vi "Format Header.vi"(5 "Name":string[](array[string]), 7 "Value":string[](array[string]), 11 "IPersist in":refnum<class "IPersist.lvclass">) -> (3 "IPersist out":refnum<class "IPersist.lvclass">, 4 "Header":string)   [LabVIEW 2019, in "IPersist.lvlib" / "IPersist.lvclass"]
uses:
  <vilib>/gpm_packages/@cs/persistence/source/IPersist/IPersist.lvclass
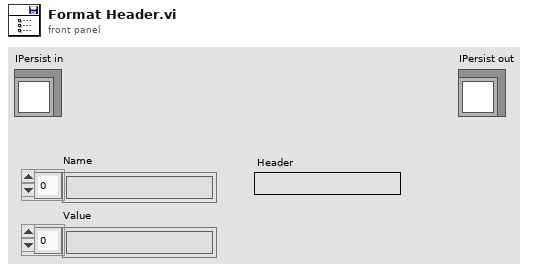
[diagram p1: front panel]
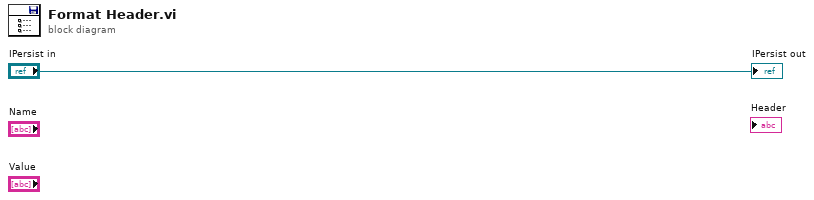
[diagram p0: block diagram]
diagram:
  "IPersist out" <- "IPersist in"
